vi "Hysteresis-GetColumnCovariance.vi"(10 "Pictures":cluster{"Fwd":dbl[][], "Bwd":dbl[][]}) -> (1 "Covariances (2D)":dbl[][](array[numeric]), 2 "Covariances (in cluster)":cluster{dbl, i32, i32}[][](array[cluster]), 3 "Size":i32)   [LabVIEW 2016]
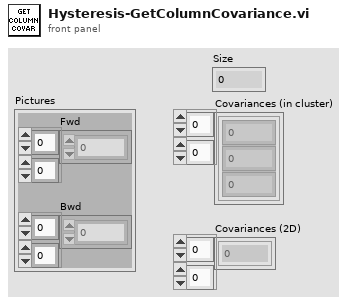
[diagram p1: front panel]
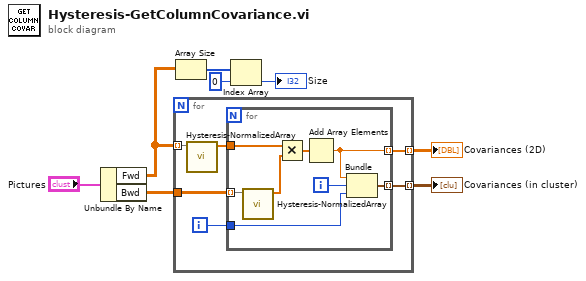
[diagram p0: block diagram]
diagram:
  n1 = Unbundle By Name("Pictures") -> ("Fwd"=w6:dbl[][], "Bwd"=w2:dbl[][])
  n2 = for {
    tunnel: w6 -> [w13] mode=indexing
    tunnel: w2 -> [w14]
    tunnel: [w11] -> w8 mode=indexing
    tunnel: [w9] -> w1 mode=indexing
    i -> [w10]
    n3 = call "Hysteresis-NormalizedArray.vi"("Array in"=w13) -> ("Array out"=w12:dbl[])  [unwired: 10 in]
    n4 = for {
      tunnel: w14 -> [w22] mode=indexing
      tunnel: w12 -> [w20]
      tunnel: w10 -> [w16]
      tunnel: [w18] -> w11 mode=indexing
      tunnel: [w17] -> w9 mode=indexing
      i -> [w15]
      n5 = call "Hysteresis-NormalizedArray.vi"("Array in"=w22) -> ("Array out"=w21:dbl[])  [unwired: 10 in]
      n6 = Multiply(x=w20, y=w21) -> (x*y=w19:dbl[])
      n7 = Add Array Elements(numeric array=w19) -> (sum=w17:dbl)
      n8 = Bundle(w17, w15, w16) -> (w18:cluster{dbl, i32, i32})  [unwired: 1 in]
    }
  }
  "Covariances (in cluster)" <- w8
  "Covariances (2D)" <- w1
  n9 = Array Size(array=w6) -> (size(s)=w5:i32[])
  n10 = Index Array(array=w5, index=0) -> (element=→"Size":i32)
